vi "SPI_Read.vi"() -> ()   [LabVIEW 2019]
uses:
  <vilib>/rvi/eio/common/nirviEmuTemplateMethod_errors.vi
  <vilib>/eio/EIONode/EIONode.xnode
panel:
  out "number":u8
  in  "bit_index":i16
  in  "rising edge":bool
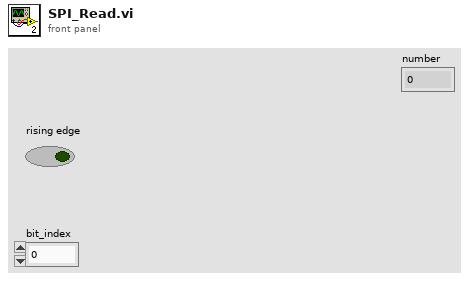
[diagram p1: front panel]
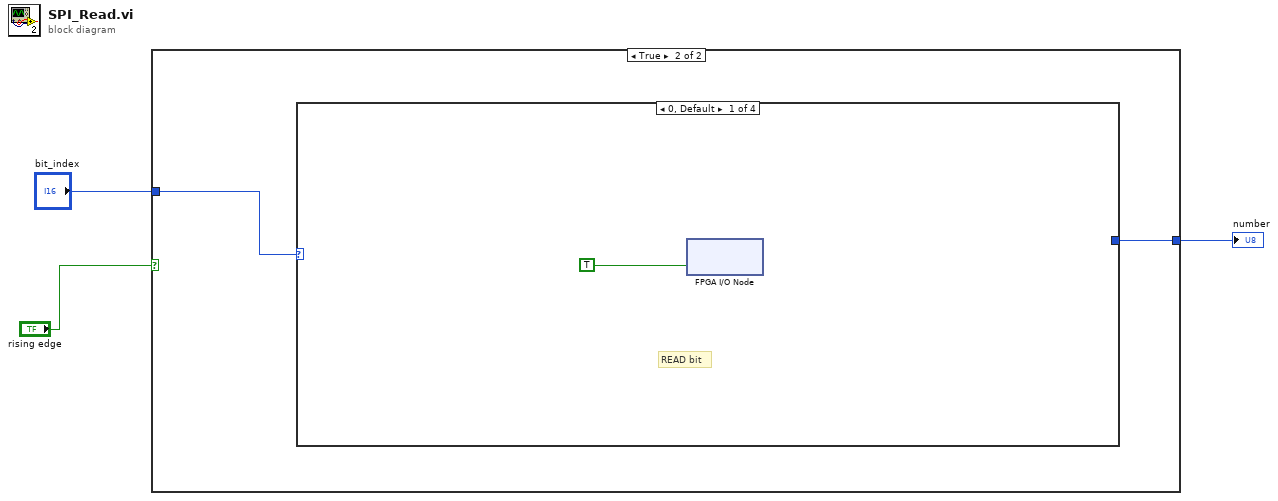
[diagram p0: block diagram]
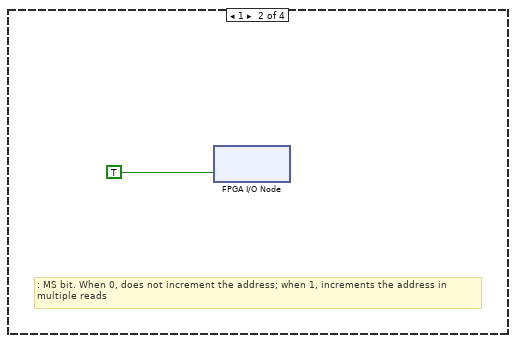
[diagram p3: hidden frame]
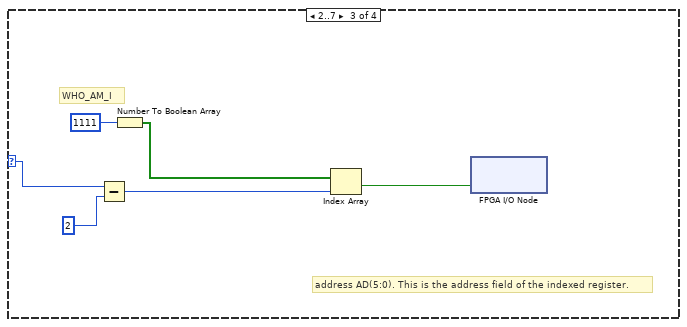
[diagram p4: hidden frame]
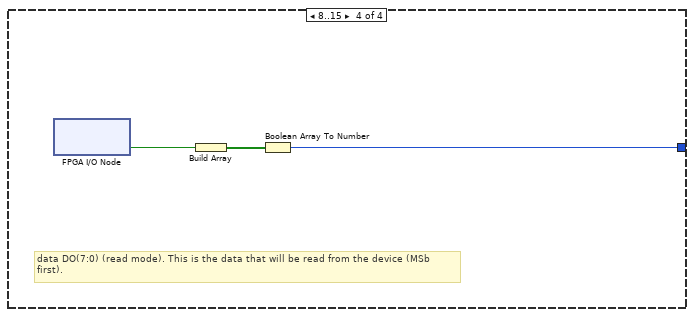
[diagram p5: hidden frame]
diagram:
  n1 = case shown="True" "rising edge" {
    tunnel: "bit_index" -> [_ w5]
    tunnel: [_ w4] -> w1
    frame False {
    }
    frame True {
      n2 = case shown="0, Default" w5 {
        selector: w5 -> [_ _ w12 _]
        tunnel: [_ _ _ w14] -> w4
        frame 0, Default {
          # "READ bit"
          n3 = xnode "FPGA I/O Node"("SDI"=TRUE) -> ()  [unwired: 1 in, 1 out]
        }
        frame 1 {
          # ": MS bit. When 0, does not increment the address; when 1, increments the address in\nmultiple reads"
          n4 = xnode "FPGA I/O Node"("SDI"=TRUE) -> ()  [unwired: 1 in, 1 out]
        }
        frame 2..7 {
          # "address AD(5:0). This is the address field of the indexed register."
          # "WHO_AM_I"
          n5 = Subtract(x=w12, y=i16 2) -> (x-y=w8:i16)
          n6 = Number To Boolean Array(number=u32 1111) -> (Boolean array=w9:bool[])
          n7 = Index Array(array=w9, index=w8) -> (element=w10:bool)
          n8 = xnode "FPGA I/O Node"("SDI"=w10) -> ()  [unwired: 1 in, 1 out]
        }
        frame 8..15 {
          # "data DO(7:0) (read mode). This is the data that will be read from the device (MSb\nfirst)."
          n9 = xnode "FPGA I/O Node"() -> ("SDO"=w16:bool)  [unwired: 1 in, 1 out]
          n10 = Build Array(w16) -> (w15:bool[])
          n11 = Boolean Array To Number(Boolean array=w15) -> (number=w14:u8)
        }
      }
    }
  }
  "number" <- w1
